vi "DriveDataAQ.vi"(8 "Reset?":bool, 10 "Manual Throttle":dbl, 11 "Manual?":bool) -> (2 "Throttle Out":dbl)   [LabVIEW 2015]
uses:
  navX-MXP Library/navX-MXP IMU.lvlib
  <vilib>/Rock Robotics/Network Tables/NT Write Number.vi
  navX-MXP Library/COMMON/TypeDefs/Data TypeDefs/navX Vector Data.ctl
panel:
  out "Raw Output Z":dbl[][](array[numeric])
  out "Raw Output Y":dbl[][](array[numeric])
  out "Valid?":bool
  out "Raw Output X":dbl[][](array[numeric])
  out "Linear Acceleration":T1
  in  "Set Throttle":dbl
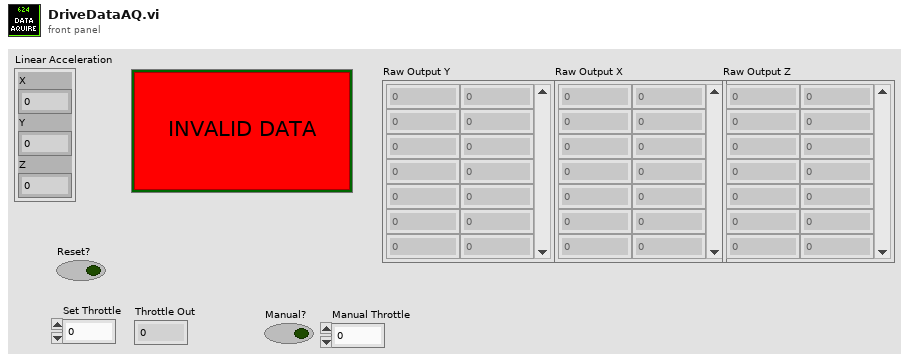
[diagram p1: front panel]
types:
  T1 = typedef "navX-MXP IMU.lvlib/navX Vector Data.ctl" = cluster{"X":dbl, "Y":dbl, "Z":dbl}
  T2 = typedef "navX-MXP IMU.lvlib/navX Device TypeDef.ctl" = cluster{"navX Interface Protocol":T3, "navX Interface Protocol TypeDefs":cluster{"SPIDevRef":T4, "I2CDevRef":T6}, "navX System Information":cluster{"Board Information":T8, "Status":T9, "Offsets":T13}, "navX Common Information":cluster{"Update Rate (4Hz-60Hz)":T14, "refnum name":string, "error":errorcluster}}
  T3 = typedef "navX-MXP IMU.lvlib/navX Interface Protocol.ctl" = enum16{"SPI", "I2C"}
  T4 = typedef "WPI_SPIDevRef.ctl" = cluster{"DevStatus":errorcluster, "Handle":i32, "SPI Bus":T5}
  T5 = typedef "spi_bus.ctl" = enum16{"SPI On-Board, CS0", "SPI On-Board, CS1", "SPI On-Board, CS2", "SPI On-Board, CS3", "SPI MXP", "Invalid"}
  T6 = typedef "WPI_I2CDevRef.ctl" = cluster{"DevStatus":errorcluster, "Device Address":u8, "Handle":i32, "I2C Bus":T7}
  T7 = typedef "i2c_bus.ctl" = enum16{"I2C On-Board", "I2C MXP", "Invalid"}
  T8 = typedef "navX-MXP IMU.lvlib/navX Board Information.ctl" = cluster{"WhoAmI (50 | 0x32)":u8, "Board Revision":u8, "Firmware Major Version":u8, "Firmware Minor Version":u8}
  T9 = typedef "navX-MXP IMU.lvlib/navX Status Data.ctl" = cluster{"Update Rate Hz":u8, "Accelerometer Full-Scale Range":u8, "Gyro Full-Scale Range":u16, "NAVX_OP_STATUS":T10, "NAVX_CAL_STATUS":T11, "NAVX_SELFTEST_STATUS":u8, "NAVX_SENSOR_STATUS":T12}
  T10 = typedef "navX-MXP IMU.lvlib/navX NAVX_OP_STATUS.ctl" = u8
  T11 = typedef "navX-MXP IMU.lvlib/navX NAVX_CAL_STATUS.ctl" = u8
  T12 = typedef "navX-MXP IMU.lvlib/navX NAVX_SENSOR_STATUS.ctl" = cluster{"MOVING":bool, "YAW_STABLE":bool, "MAG_DISTURBANCE":bool, "ALTITUDE_VALID":bool, "SEALEVEL_PRESS_SET":bool, "FUSED_HEADING_VALID":bool}
  T13 = typedef "navX-MXP IMU.lvlib/navX Offsets Data.ctl" = cluster{"Yaw":dbl, "Quat W":dbl, "Quat X":dbl, "Quat Y":dbl, "Quat Z":dbl}
  T14 = typedef "navX-MXP IMU.lvlib/navX Update Rate.ctl" = u8
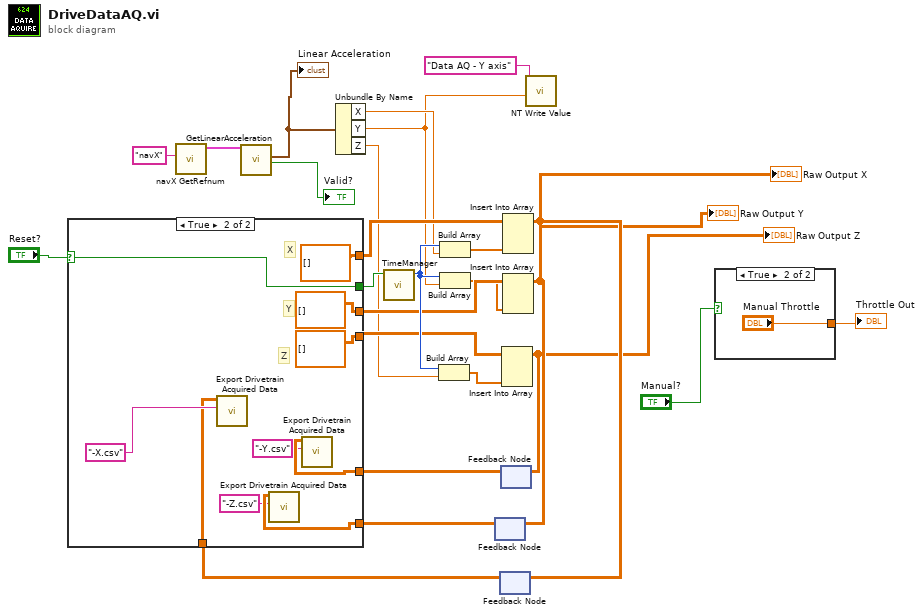
[diagram p0: block diagram]
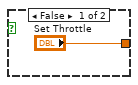
[diagram p2: hidden frame]
diagram:
  n1 = call "navX GetRefnum.vi"("refnum name"="navX") -> ("navX Device TypeDef"=w20:T2)  [unwired: 9 in, 1 out]
  n2 = call "GetLinearAcceleration.vi"("navX Device TypeDef"=w20) -> ("Valid?"=→"Valid?":bool, "Linear Acceleration"=w10:T1)  [unwired: 8 in, 1 out]
  "Linear Acceleration" <- w10
  n3 = Unbundle By Name(w10) -> ("X"=w4:dbl, "Y"=w2:dbl, "Z"=w5:dbl)
  n4 = feedback #1() -> (w13:dbl[][])  [unwired: 1 in]
  n5 = feedback #2() -> (w24:dbl[][])  [unwired: 1 in]
  n6 = feedback #3() -> (w12:dbl[][])  [unwired: 1 in]
  n7 = case shown="True" "Reset?" {
    selector: "Reset?" -> [w28 w38]
    tunnel: [w29 dbl[][] []] -> w25
    tunnel: w24 -> [w29 w34]
    tunnel: [w28 w38] -> w22
    tunnel: [w27 dbl[][] []] -> w17
    tunnel: [w26 dbl[][] []] -> w16
    tunnel: w13 -> [w27 w31]
    tunnel: w12 -> [w26 w33]
    frame False {
    }
    frame True {
      # "Z"
      # "Y"
      # "X"
      n8 = call "Export Drivetrain Acquired Data.vi"("string"="-X.csv", "Array"=w34) -> ()  [unwired: 10 in]
      n9 = call "Export Drivetrain Acquired Data.vi"("string"="-Z.csv", "Array"=w31) -> ()  [unwired: 10 in]
      n10 = call "Export Drivetrain Acquired Data.vi"("string"="-Y.csv", "Array"=w33) -> ()  [unwired: 10 in]
    }
  }
  n11 = call "TimeManager.vi"(11:w22) -> ("Time Since Reset"=w18:u32)  [unwired: 9 in, 1 out]
  n12 = Build Array(w18, w5) -> (w15:dbl[])
  n13 = Build Array(w18, w4) -> (w21:dbl[])
  n14 = Build Array(w18, w2) -> (w14:dbl[])
  n15 = Insert Into Array(array=w16, new element=w15) -> (w6:dbl[][])  [unwired: 2 in]
  "Raw Output Z" <- w6
  n16 = feedback-in #3(w6) -> ()
  n17 = Insert Into Array(array=w25, new element=w21) -> (w8:dbl[][])  [unwired: 2 in]
  "Raw Output X" <- w8
  n18 = feedback-in #2(w8) -> ()
  n19 = Insert Into Array(array=w17, new element=w14) -> (w7:dbl[][])  [unwired: 2 in]
  "Raw Output Y" <- w7
  n20 = feedback-in #1(w7) -> ()
  n21 = call-poly <vilib>:"NT Write Value.vi"("Numeric"=w2, "Name"="Data AQ - Y axis") -> ()  [unwired: 9 in, 1 out]
  n22 = case shown="True" "Manual?" {
    tunnel: ["Set Throttle" "Manual Throttle"] -> w11
    frame False {
    }
    frame True {
    }
  }
  "Throttle Out" <- w11
